vi "getEventInternalCommand.vi"(8 "error in (no error)":errorcluster, 11 "SALCommunicatorController in":refnum<class "SALCommunicatorController.lvclass">) -> (0 "error out":errorcluster, 1 "function return":i32, 2 "logevent_InternalCommand_Ctl out":T1, 3 "SALCommunicatorController out":refnum<class "SALCommunicatorController.lvclass">)   [LabVIEW 2016, in "SALCommunicatorController.lvclass"]
uses:
  SALCommunicatorController.lvclass
  ts_sallv_exa/DataTypes/logevent_InternalCommand.ctl
  ts_sallv_exa/SALLV_EXA.lvlib
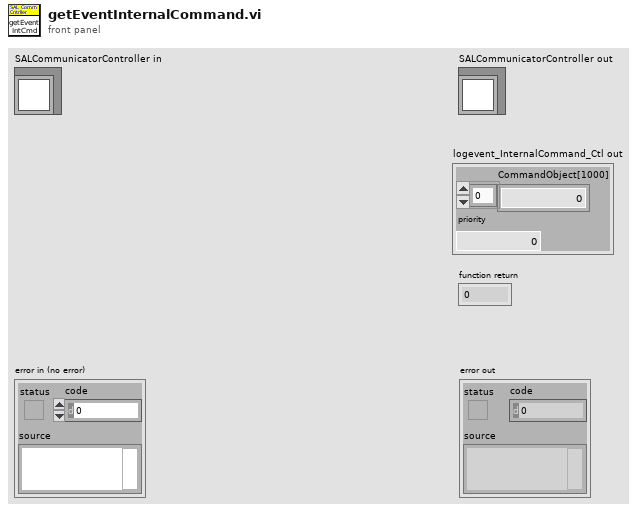
[diagram p1: front panel]
types:
  T1 = typedef "SALLV_EXA.lvlib/logevent_InternalCommand.ctl" = cluster{"CommandObject[1000]":u8[], "priority":i32}
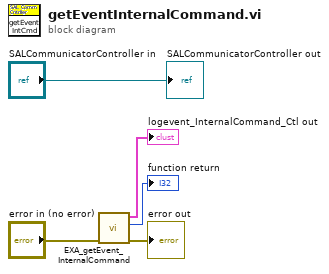
[diagram p0: block diagram]
diagram:
  n1 = call "EXA_getEvent_InternalCommand.vi"("error in (no error)"="error in (no error)") -> ("error out"=→"error out":errorcluster, "function return"=→"function return":i32, "logevent_InternalCommand_Ctl out"=→"logevent_InternalCommand_Ctl out":T1)  [unwired: 8 in]
  "SALCommunicatorController out" <- "SALCommunicatorController in"
